vi "PID Normalize Step.vi"(0 "stimulus signal":dbl[](array[numeric]), 1 "with initial part?":bool, 5 "response signal":dbl[](array[numeric])) -> (2 "stimulus offset":dbl, 3 "Start index":i32, 4 "response norm":dbl[](array[numeric]), 6 "length":i32, 10 "noise":dbl, 13 "response offset":dbl, 14 "K":dbl, 15 "error code":i32)   [LabVIEW 2017, in "NI_PID_autopid.lvlib"]
uses:
  <vilib>/addons/control/pid/NI_PID_autopid.lvlib
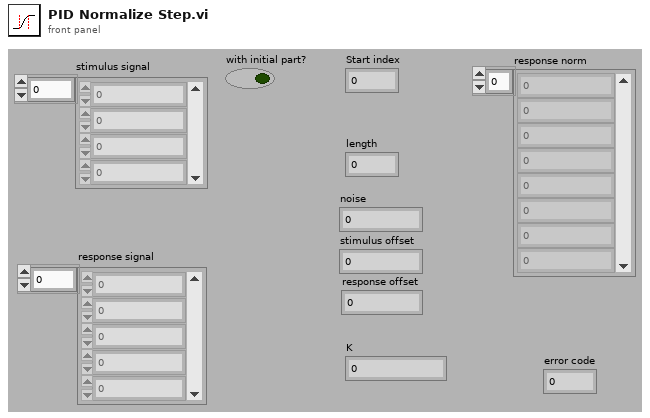
[diagram p1: front panel]
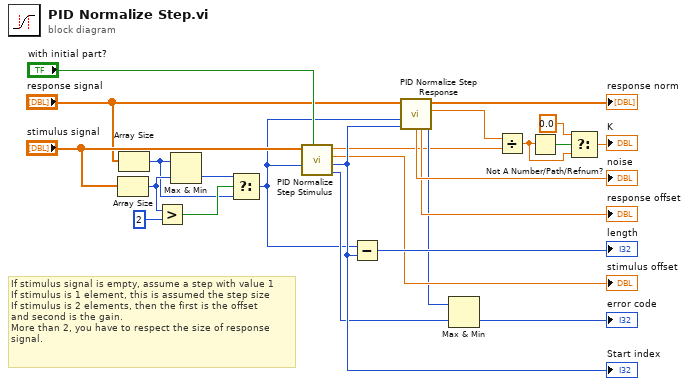
[diagram p0: block diagram]
diagram:
  # "If stimulus signal is empty, assume a step with value 1\nIf stimulus is 1 element, this is assumed the step size\nIf stimulus is 2 elements, then the first is the offset \nand second is the gain.\nMore than 2, you have to respect the size of response\nsignal."
  n1 = Array Size(array="stimulus signal") -> (size(s)=w6:i32)
  n2 = Array Size(array="response signal") -> (size(s)=w3:i32)
  n3 = Greater?(x=w6, y=2) -> (0:w4:bool)
  n4 = Max & Min(x=w3, y=w6) -> (min(x,y)=w2:i32)  [unwired: 1 out]
  n5 = Select(t=w2, s=w4, f=w3) -> (s? t:f=w1:i32)
  n6 = call <vilib>:"PID Normalize Step Stimulus.vi"("with initial part?"="with initial part?", "Length"=w1, "Stimulus signal"="stimulus signal") -> ("error code"=w14:i32, "Index for start step"=w21:i32, "Offset"=→"stimulus offset":dbl, "Step height"=w11:dbl)  [unwired: 5 in]
  "Start index" <- w21
  n7 = Subtract(x=w1, y=w21) -> (x-y=→"length":i32)
  n8 = call <vilib>:"PID Normalize Step Response.vi"("start index"=w21, "length"=w1, "response signal"="response signal") -> ("error code"=w13:i32, "noise"=→"noise":dbl, "step height"=w12:dbl, "response norm"=→"response norm":dbl[], "response offset"=→"response offset":dbl)  [unwired: 4 in]
  n9 = Max & Min(x=w13, y=w14) -> (min(x,y)=→"error code":i32)  [unwired: 1 out]
  n10 = Divide(x=w12, y=w11) -> (x/y=w7:dbl)
  n11 = Not A Number/Path/Refnum?(number/path/refnum=w7) -> (NaN/Path/Refnum?=w10:bool)
  n12 = Select(t=0.0 ("f"), s=w10, f=w7) -> (s? t:f=→"K":dbl)
